vi "ScurrDataIn.vi"(7 "测试类型":string, 8 "error in (no error)":errorcluster, 9 "温度":dbl, 10 "Vout":dbl, 11 "通道":u16(ring) items=["CH1", "CH2", "CH3", "CH4", "CH5", "CH6", "CH7", "CH8"]) -> (0 "error out":errorcluster)   [LabVIEW 2014]
panel:
  in  "数组":dbl[](array[numeric])=[12.0, 12.0, 6.4, 2.2, 5.1, 5.0, 17.8]
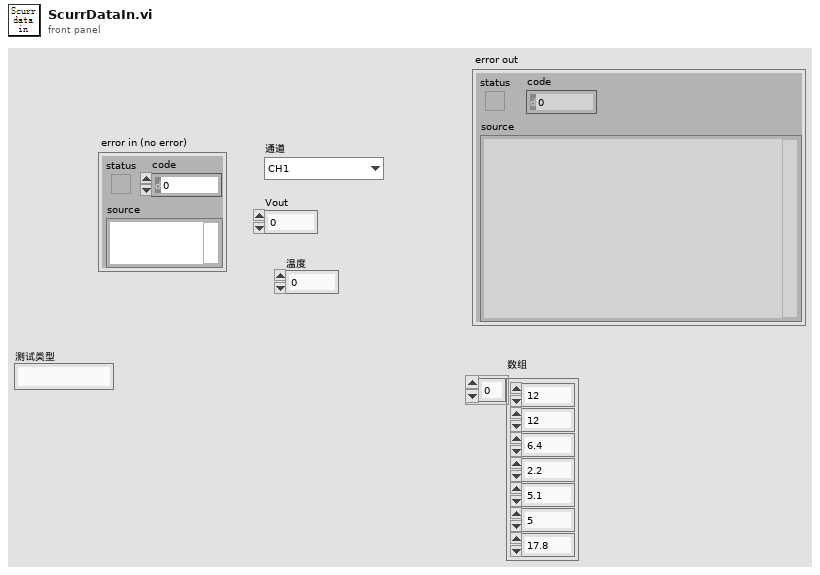
[diagram p1: front panel]
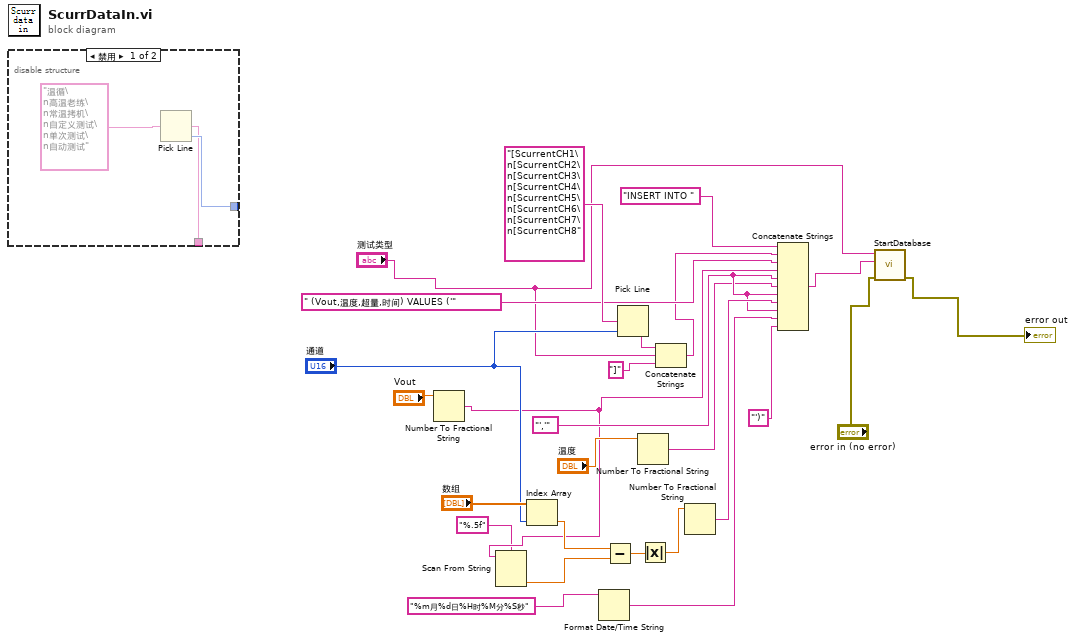
[diagram p0: block diagram]
diagram:
  w17 = "','"
  n1 = disable-structure shown="禁用" {
    disable-tunnel: _ -> [w28 _]
    disable-tunnel: [w27 _] -> _
    frame Disabled {
      n2 = Pick Line(multi-line string="温循\n高温老练\n常温拷机\n自定义测试\n单次测试\n自动测试" ("多行字符串"), line index=w28) -> (output string=w27:string)  [unwired: 1 in]
    }
    frame Enabled {
    }
  }
  n3 = Number To Fractional String(number="Vout") -> (F-format string=w3:string)  [unwired: 3 in]
  n4 = Scan From String(format string="%.5f" ("格式字符串"), input string=w3) -> (output 1=w1:dbl)  [unwired: 3 in, 3 out]
  n5 = Index Array(array="数组", index="通道") -> (element=w23:dbl)
  n6 = Format Date/Time String(time format string (%c)="%m月%d日%H时%M分%S秒" ("时间格式字符串(%c)")) -> (date/time string=w16:string)  [unwired: 2 in]
  n7 = Subtract(x=w23, y=w1) -> (x-y=w22:dbl)
  n8 = Pick Line(multi-line string="[ScurrentCH1\n[ScurrentCH2\n[ScurrentCH3\n[ScurrentCH4\n[ScurrentCH5\n[ScurrentCH6\n[ScurrentCH7\n[ScurrentCH8" ("多行字符串"), line index="通道") -> (output string=w9:string)  [unwired: 1 in]
  n9 = Number To Fractional String(number="温度") -> (F-format string=w6:string)  [unwired: 3 in]
  n10 = Absolute Value(x=w22) -> (abs(x)=w14:dbl)
  n11 = Concatenate Strings(w9, "测试类型", "]") -> (w10:string)
  n12 = Number To Fractional String(number=w14) -> (F-format string=w18:string)  [unwired: 3 in]
  n13 = Concatenate Strings("INSERT INTO ", w10, " (Vout,温度,超量,时间) VALUES ('", w3, w17, w6, w17, w18, w17, w16, "')") -> (w13:string)
  n14 = call "StartDatabase.vi"("error in (no error)"="error in (no error)", "SQL query"=w13, "测试类型"="测试类型") -> ("error out 2"=→"error out":errorcluster)  [unwired: 8 in]
